vi "Default Delay Time.vi"(8 "error in (no error)":errorcluster) -> (0 "error out":errorcluster, 3 "Delay Time":dbl[](array[numeric]) format="%#_6p")   [LabVIEW 2020]
uses:
  <vilib>/Utility/config.llb/Read Key (Double).vi
  Labview Library/Libraries/UT_Utilities/Utilities.lvlib
  <vilib>/Utility/config.llb/NI_LVConfig.lvlib
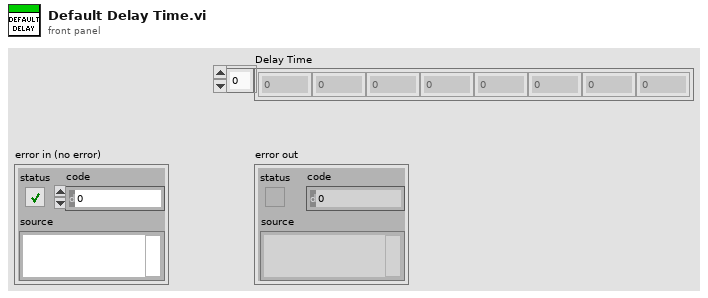
[diagram p1: front panel]
types:
  T1 = typedef "NI_LVConfig.lvlib/Config Data RefNum.ctl" = refnum<k1>
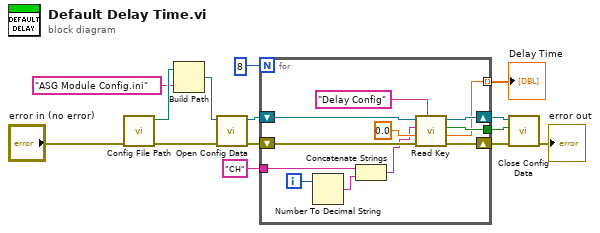
[diagram p0: block diagram]
diagram:
  n1 = call "Config File Path.vi"("error in (no error)"="error in (no error)") -> ("error out"=w12:errorcluster, "Config File Path"=w10:path)  [unwired: 9 in]
  n2 = Build Path(base path=w10, name or relative path="ASG Module Config.ini") -> (appended path=w11:path)
  n3 = call <vilib>:"Open Config Data.vi"("error in (no error)"=w12, "configuration file path"=w11) -> ("error out"=w14:errorcluster, "refnum"=w13:T1)  [unwired: 7 in, 1 out]
  n4 = for {
    N: 8 -> [_]
    tunnel: [w22] -> w6
    shift-right: [w23] -> w7
    shift-left: w14 -> [w26]
    shift-right: [w21] -> w5
    shift-left: w13 -> [w25]
    tunnel: "CH" ("key") -> [w17]
    tunnel: [w16] -> w2 mode=indexing
    i -> [w19]
    n5 = Number To Decimal String(number=w19) -> (decimal integer string=w18:string)  [unwired: 1 in]
    n6 = Concatenate Strings(w17, w18) -> (w15:string)
    n7 = call-poly <vilib>:"Read Key.vi"("section"="Delay Config", "error in (no error)"=w26, "default value"=0.0, "key"=w15, "refnum"=w25) -> ("error out"=w23:errorcluster, "value"=w16:dbl, "found?"=w22:bool, "refnum out"=w21:T1)  [unwired: 3 in]
  }
  "Delay Time" <- w2
  n8 = call <vilib>:"Close Config Data.vi"("error in (no error)"=w7, "write file if changed (T)"=w6, "refnum"=w5) -> ("error out"=→"error out":errorcluster)  [unwired: 7 in, 1 out]
